vi "Alicat read setpoint.vi"(3 "Unit ID":string="P", 5 "ALICAT COM Port":refnum<visa-resource-name>="COM5") -> (1 "Measurement Data":T1)   [LabVIEW 2023]
panel:
  out "Error Text":string
  out "Range Exceeded":bool
  out "Error Present":bool
  # "Totalizer Timer"
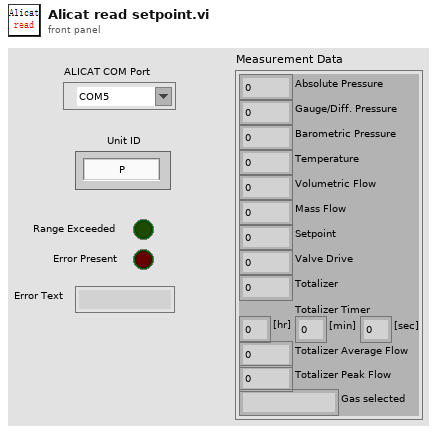
[diagram p1: front panel]
types:
  T1 = cluster{"Absolute Pressure":dbl, "Gauge/Diff. Pressure":dbl, "Barometric Pressure":dbl, "Temperature":dbl, "Volumetric Flow":dbl, "Mass Flow":dbl, "Setpoint":dbl, "Valve Drive":dbl, "Totalizer":dbl, "[hr]":dbl, "[min]":dbl, "[sec]":dbl, "Totalizer Average Flow":dbl, "Totalizer Peak Flow":dbl, "Gas selected":string}
  T2 = enum8{"2400", "9600", "19200", "38400", "57600", "115200", "Unknown"}
  T3 = cluster{"Unit ID":string, "Baud Rate":enum8{"2400", "9600", "19200", "38400", "57600", "115200", "Unknown"}, "ALICAT COM Port":refnum<visa-resource-name>}
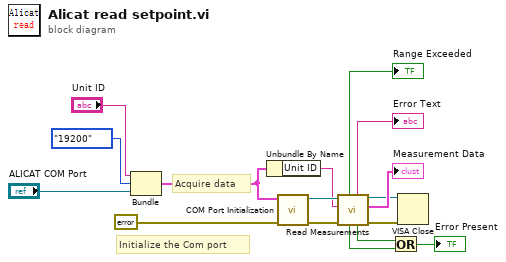
[diagram p0: block diagram]
diagram:
  # "Initialize the Com port"
  # "Acquire data"
  n1 = Bundle("Unit ID"="Unit ID", "Baud Rate"=T2."19200", "ALICAT COM Port"="ALICAT COM Port") -> (w3:T3)  [unwired: 1 in]
  n2 = Unbundle By Name(w3) -> ("Unit ID"=w12:string)
  n3 = call "COM Port Initialization.vi"("error in (no error)"=errorcluster {"status"=FALSE, "code"=0, "source"=""}, "Communication Settings"=w3) -> ("error out"=w14:errorcluster, "VISA Session Out"=w15:refnum<visa-resource-name>)  [unwired: 8 in]
  n4 = call "Read Measurements.vi"("error in"=w14, "Unit ID (A)"=w12, "VISA Session In"=w15) -> ("error out"=w2:errorcluster, "Data Cluster"=→"Measurement Data":T1, "VISA Session Out"=w1:refnum<visa-resource-name>, "Unknown Dataframe Info"=w10:bool, "Error/Overrange/Unknown String"=→"Error Text":string, "Error Present"=w9:bool, "Range Exceeded"=→"Range Exceeded":bool)  [unwired: 1 in, 1 out]
  n5 = Or(x=w10, y=w9) -> (x .or. y?=→"Error Present":bool)
  n6 = VISA Close(VISA resource name=w1, error in (no error)=w2) -> ()  [unwired: 1 out]
